vi "example_2_8_a.vi"() -> ()   [LabVIEW 2018]
panel:
  out "XY Graph":cluster{dbl[], u16[]}(graph)
  in  "stop":bool
  out "Area":dbl format="%.2f"
  in  "Base":u16
  in  "Altitude":u16
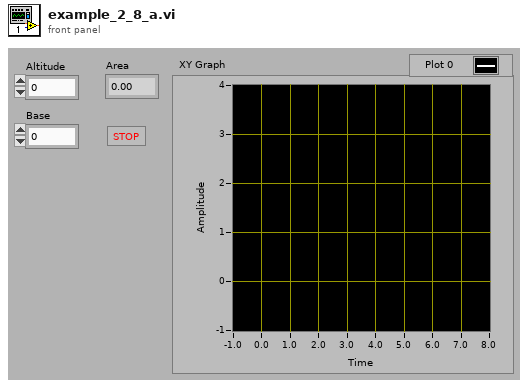
[diagram p1: front panel]
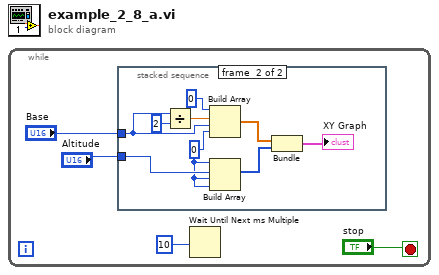
[diagram p0: block diagram]
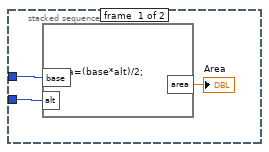
[diagram p2: hidden frame]
diagram:
  n1 = while {
    stop <- "stop" stop-if-true
    n2 = stacked-sequence {
      tunnel: "Base" -> [w7 w11]
      tunnel: "Altitude" -> [w6 w10]
      frame #0 {
        n3 = formula code="area=(base*alt)/2;"("base"=w7, "alt"=w6) -> ("area"=→"Area":dbl)
      }
      frame #1 {
        w8 = u16 0 ("Input Element")
        n4 = Divide(x=w11, y=u16 2) -> (x/y=w9:dbl)
        n5 = Build Array(u16 0 ("Input Element"), w9, w11, w8) -> (w16:dbl[])
        n6 = Build Array(w8, w10, w8, w8) -> (w14:u16[])
        n7 = Bundle(w16, w14) -> (→"XY Graph":cluster{dbl[], u16[]})  [unwired: 1 in]
      }
    }
    n8 = Wait Until Next ms Multiple(millisecond multiple=u32 10 ("milliseconds to wait")) -> ()  [unwired: 1 out]
  }
